vi "perm_comb.vi"() -> ()   [LabVIEW 2023]
panel:
  out "C":dbl
  out "P":dbl
  in  "R":dbl
  in  "N":dbl
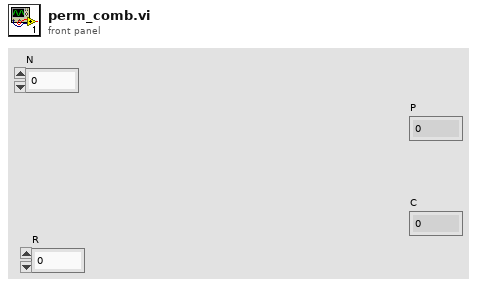
[diagram p1: front panel]
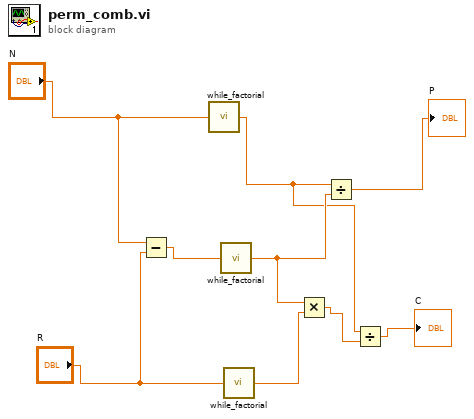
[diagram p0: block diagram]
diagram:
  n1 = Subtract(x="N", y="R") -> (x-y=w6:dbl)
  n2 = call "while_factorial.vi"("Number"="N") -> ("Factorial"=w1:dbl)
  n3 = call "while_factorial.vi"("Number"=w6) -> ("Factorial"=w5:dbl)
  n4 = call "while_factorial.vi"("Number"="R") -> ("Factorial"=w4:dbl)
  n5 = Multiply(x=w5, y=w4) -> (x*y=w3:dbl)
  n6 = Divide(x=w1, y=w5) -> (x/y=→"P":dbl)
  n7 = Divide(x=w1, y=w3) -> (x/y=→"C":dbl)
